vi "USB2XXX_LINEX_MasterTest.vi"() -> ()   [LabVIEW 2010]
uses:
  PublicFiles/USB2XXX.dll
panel:
  in  "stop":bool
  in  "Excute":bool
  in  "pInMsg 3":T1={"Timestamp"=20, "MsgType"=2, "CheckType"=0, "DataLen"=8, "Sync"=85, "PID"=3, "Data[0]"=33, "Data[1]"=34, "Data[2]"=35, "Data[3]"=36, "Data[4]"=37, "Data[5]"=38, "Data[6]"=39, "Data[7]"=40, "Check"=1, "Reserve"=0, "Reserve"=0} {"Sync" format="%x"; "PID" format="%x"; "Data[0]" format="%x"; "Data[1]" format="%x"; "Data[2]" format="%x"; "Data[3]" format="%x"; "Data[4]" format="%x"; "Data[5]" format="%x"; "Data[6]" format="%x"; "Data[7]" format="%x"; "Check" format="%x"; "Reserve" format="%x"; "Reserve" format="%x"}
  in  "pInMsg 2":T1={"Timestamp"=20, "MsgType"=2, "CheckType"=0, "DataLen"=8, "Sync"=85, "PID"=2, "Data[0]"=17, "Data[1]"=18, "Data[2]"=19, "Data[3]"=20, "Data[4]"=21, "Data[5]"=22, "Data[6]"=23, "Data[7]"=24, "Check"=1, "Reserve"=0, "Reserve"=0} {"Sync" format="%x"; "PID" format="%x"; "Data[0]" format="%x"; "Data[1]" format="%x"; "Data[2]" format="%x"; "Data[3]" format="%x"; "Data[4]" format="%x"; "Data[5]" format="%x"; "Data[6]" format="%x"; "Data[7]" format="%x"; "Check" format="%x"; "Reserve" format="%x"; "Reserve" format="%x"}
  out "pOutMsg":T2(array[cluster]) {"Sync" format="%x"; "PID" format="%x"; "Data[0]" format="%x"; "Data[1]" format="%x"; "Data[2]" format="%x"; "Data[3]" format="%x"; "Data[4]" format="%x"; "Data[5]" format="%x"; "Data[6]" format="%x"; "Data[7]" format="%x"; "Check" format="%x"}
  in  "pInMsg":T1={"Timestamp"=20, "MsgType"=1, "CheckType"=0, "DataLen"=8, "Sync"=85, "PID"=1, "Data[0]"=1, "Data[1]"=2, "Data[2]"=3, "Data[3]"=4, "Data[4]"=5, "Data[5]"=6, "Data[6]"=7, "Data[7]"=8, "Check"=1, "Reserve"=0, "Reserve"=0} {"Sync" format="%x"; "PID" format="%x"; "Data[0]" format="%x"; "Data[1]" format="%x"; "Data[2]" format="%x"; "Data[3]" format="%x"; "Data[4]" format="%x"; "Data[5]" format="%x"; "Data[6]" format="%x"; "Data[7]" format="%x"; "Check" format="%x"; "Reserve" format="%x"; "Reserve" format="%x"}
  out "function return":i32
  in  "BaudRate":u32=19200
  in  "Channel Index":u8(ring) items=["CH0"]
  in  "Device Index":i32(ring) items=["0", "1", "2", "3", "4", "5"]
  # "波特率一定要设置，否则程序可能出错"
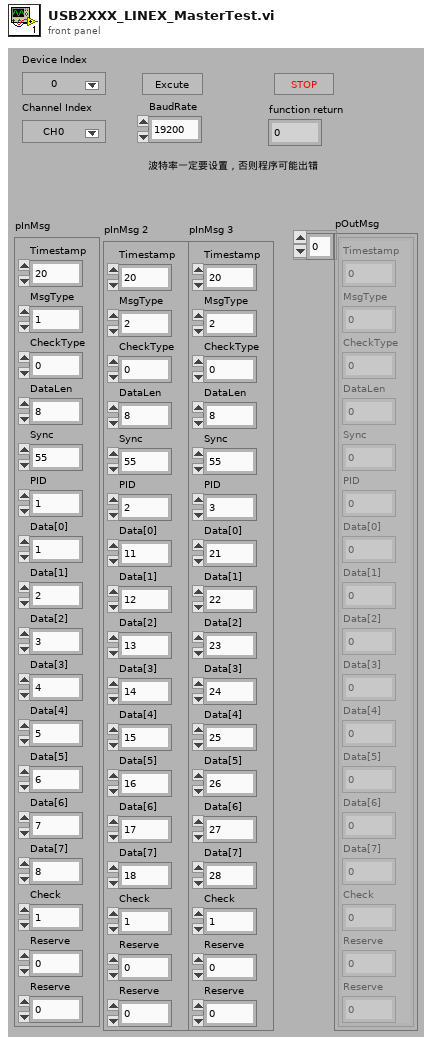
[diagram p1: front panel]
types:
  T1 = cluster{"Timestamp":u32, "MsgType":u8, "CheckType":u8, "DataLen":u8, "Sync":u8, "PID":u8, "Data[0]":u8, "Data[1]":u8, "Data[2]":u8, "Data[3]":u8, "Data[4]":u8, "Data[5]":u8, "Data[6]":u8, "Data[7]":u8, "Check":u8, "Reserve":u8, "Reserve":u8}
  T2 = cluster{"Timestamp":u32, "MsgType":u8, "CheckType":u8, "DataLen":u8, "Sync":u8, "PID":u8, "Data[0]":u8, "Data[1]":u8, "Data[2]":u8, "Data[3]":u8, "Data[4]":u8, "Data[5]":u8, "Data[6]":u8, "Data[7]":u8, "Check":u8, "Reserve":u8, "Reserve":u8}[]
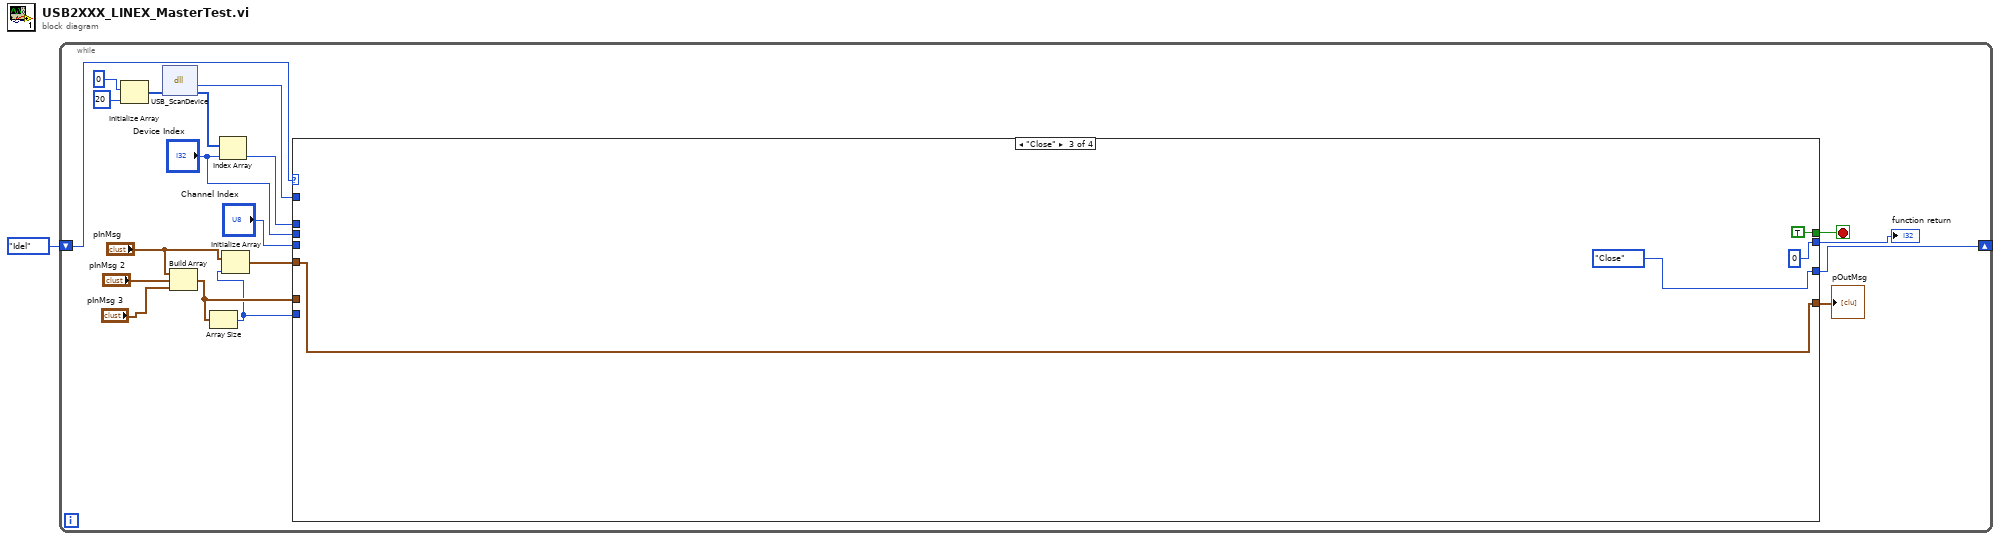
[diagram p0: block diagram]
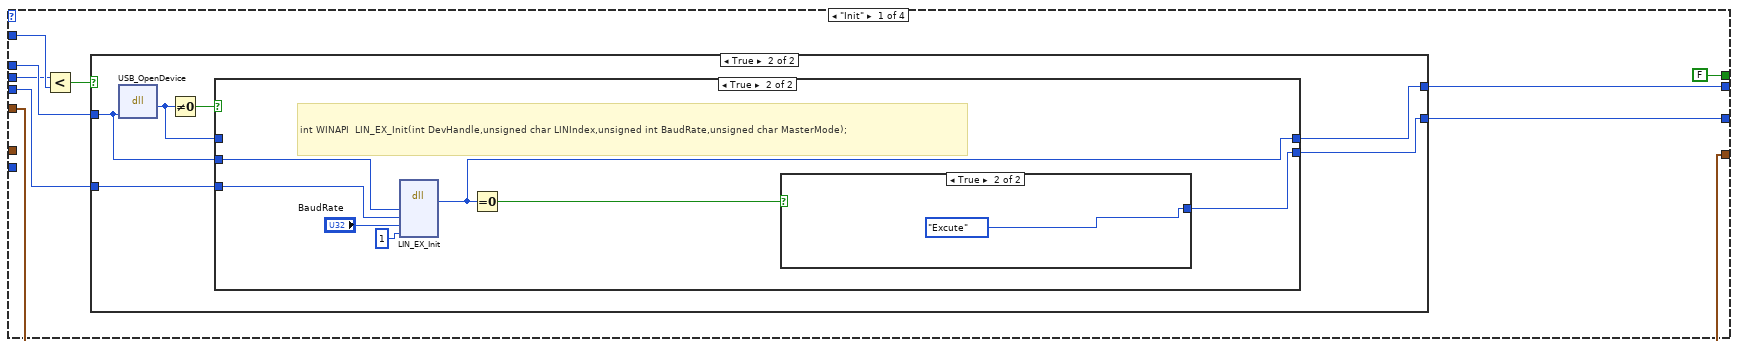
[diagram p2: hidden frame]
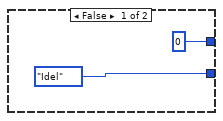
[diagram p3: hidden frame]
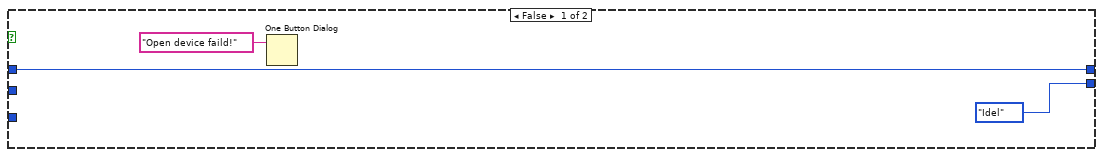
[diagram p4: hidden frame]
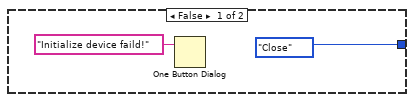
[diagram p5: hidden frame]
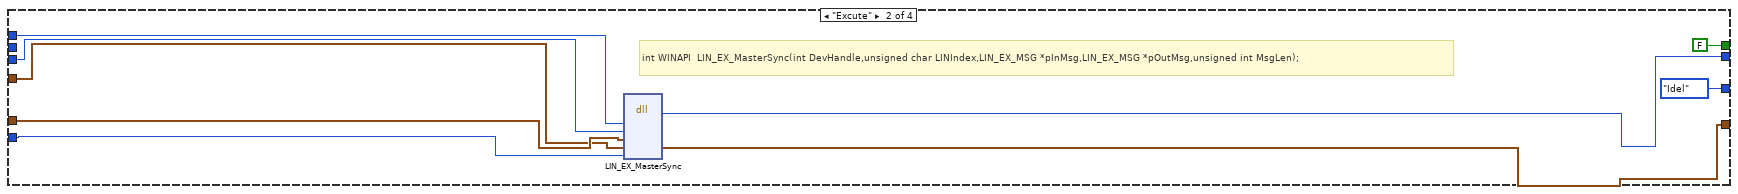
[diagram p6: hidden frame]
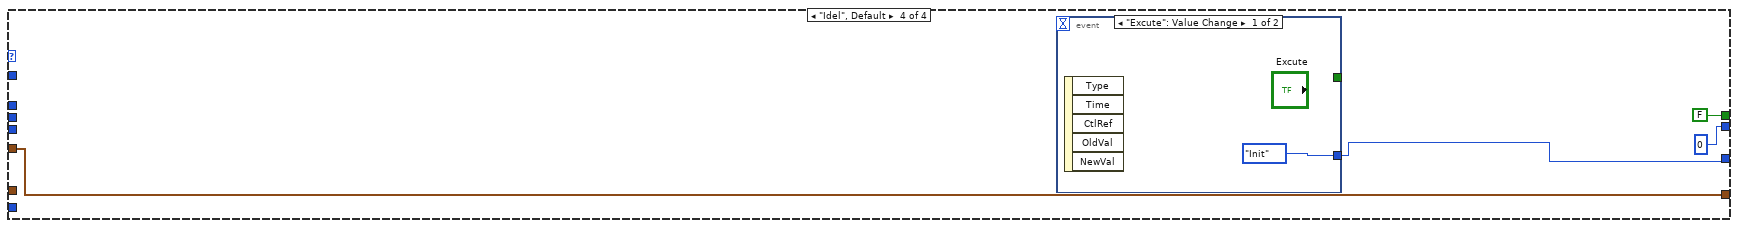
[diagram p7: hidden frame]
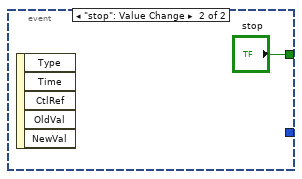
[diagram p8: hidden frame]
diagram:
  n1 = while {
    shift-right: [w19] -> _
    shift-left: enum16{"Init", "Excute", "Idel", "Close"}."Idel" ("Enum") -> [w20]
    stop <- w17 stop-if-true
    n2 = Initialize Array(0, 20 ("dimension size")) -> (w16:i32[])
    n3 = dll-call lib="E:/OtherWork/STM32/USB2XXX_Example/examples/Labview/PublicFiles/USB2XXX.dll" fn="USB_ScanDevice"("pDevNum"=w16) -> ("return type"=w12:i32, "pDevNum"=w13:i32[])  [unwired: 3 in, 2 out]
    n4 = Build Array("pInMsg", "pInMsg 2", "pInMsg 3") -> (w3:T2)
    n5 = Array Size(array=w3) -> (size(s)=w2:i32)
    n6 = Index Array(array=w13, index="Device Index") -> (element=w7:i32)
    n7 = Initialize Array("pInMsg", w2) -> (w10:T2)
    n8 = case shown="\"Close\"" w20 {
      tunnel: [w28 enum16{"Init", "Excute", "Idel", "Close"}."Idel" ("Enum") enum16{"Init", "Excute", "Idel", "Close"}."Close" ("Enum") w64] -> w19
      tunnel: w7 -> [w24 w57 _ _]
      tunnel: "Channel Index" -> [w27 w56 _ _]
      tunnel: [FALSE FALSE TRUE FALSE] -> w17
      tunnel: w12 -> [w25 _ _ _]
      tunnel: "Device Index" -> [w23 _ _ _]
      tunnel: w2 -> [_ w55 _ _]
      tunnel: w10 -> [w22 w53 w63 w66]
      tunnel: w3 -> [_ w54 _ _]
      tunnel: [w22 w51 w63 w66] -> w9
      tunnel: [w21 w52 0 ("return type") 0 ("return type")] -> w8
      frame "Init" {
        n9 = Less?(x=w23, y=w25) -> (x < y?=w29:bool)
        n10 = case shown="True" w29 {
          tunnel: w24 -> [_ w35]
          tunnel: w27 -> [_ w36]
          tunnel: [enum16{"Init", "Excute", "Idel", "Close"}."Idel" ("Enum") w34] -> w28
          tunnel: [0 ("return type") w33] -> w21
          frame False {
          }
          frame True {
            n11 = dll-call lib="E:/OtherWork/STM32/USB2XXX_Example/examples/Labview/PublicFiles/USB2XXX.dll" fn="USB_OpenDevice"("DevIndex"=w35) -> ("return type"=w32:u8)  [unwired: 4 in, 2 out]
            n12 = Not Equal To 0?(x=w32) -> (x != 0?=w37:bool)
            n13 = case shown="True" w37 {
              tunnel: w36 -> [_ w43]
              tunnel: w35 -> [_ w44]
              tunnel: [enum16{"Init", "Excute", "Idel", "Close"}."Idel" ("Enum") w46] -> w34
              tunnel: [w39 w41] -> w33
              tunnel: w32 -> [w39 _]
              frame False {
                n14 = One Button Dialog(message="Open device faild!") -> ()  [unwired: 1 in, 1 out]
              }
              frame True {
                # "int WINAPI  LIN_EX_Init(int DevHandle,unsigned char LINIndex,unsigned int BaudRate,unsigned char MasterMode);"
                n15 = dll-call lib="E:/OtherWork/STM32/USB2XXX_Example/examples/Labview/PublicFiles/USB2XXX.dll" fn="LIN_EX_Init"("DevHandle"=w44, "LINIndex"=w43, "BaudRate"="BaudRate", "MasterMode"=u8 1) -> ("return type"=w41:i32)  [unwired: 7 in, 2 out]
                n16 = Equal To 0?(x=w41) -> (x = 0?=w47:bool)
                n17 = case shown="True" w47 {
                  tunnel: [enum16{"Init", "Excute", "Idel", "Close"}."Close" ("Enum") enum16{"Init", "Excute", "Idel", "Close"}."Excute" ("Enum")] -> w46
                  frame False {
                    n18 = One Button Dialog(message="Initialize device faild!") -> ()  [unwired: 1 in, 1 out]
                  }
                  frame True {
                  }
                }
              }
            }
          }
        }
      }
      frame "Excute" {
        # "int WINAPI  LIN_EX_MasterSync(int DevHandle,unsigned char LINIndex,LIN_EX_MSG *pInMsg,LIN_EX_MSG *pOutMsg,unsigned int MsgLen);"
        n19 = dll-call lib="E:/OtherWork/STM32/USB2XXX_Example/examples/Labview/PublicFiles/USB2XXX.dll" fn="LIN_EX_MasterSync"("DevHandle"=w57, "LINIndex"=w56, "pInMsg"=w54, "pOutMsg"=w53, "MsgLen"=w55) -> ("return type"=w52:i32, "pOutMsg"=w51:T2)  [unwired: 7 in, 2 out]
      }
      frame "Close" {
      }
      frame "Idel", Default {
        n20 = event shown="[0] \"Excute\": Value Change" {
          selector: _ -> [_ _]
          dyn-events: _ -> [_ _]
          timeout: _ -> [_ _]
          tunnel: [_ "stop"] -> _
          tunnel: [enum16{"Init", "Excute", "Idel", "Close"}."Init" ("Enum") _] -> w64
          event "Excute": Value Change {
            n21 = event-data() -> ()  [unwired: 1 in, 5 out]
          }
          event "stop": Value Change {
            n22 = event-data() -> ()  [unwired: 1 in, 5 out]
          }
        }
      }
    }
    "pOutMsg" <- w9
    "function return" <- w8
  }
